vi "MGCC_StaEst_main_HTB.vi"() -> ()   [LabVIEW 2016]
doc: "This VI is designed for the state estimation function block. The current version is designed for IEEE13node system. The advanced model will be available in the latest version. There is no input for this VI. Bascially, the input right now comes from the cvs in IEEE13 folder."
uses:
  Finite State Machine/Sub-VIs/MGCC_FntStaMach_gobal.vi
  <vilib>/imath/engines/lvmath2/RunTimeEngine/IndexRead/NIMS M(S,$).vi
  <instcachedir>/0/NIMS M(S,$)_F24F360562DE41D8BE234322A2E15C65.lvgen/NIMS M(S,$)_F24F360562DE41D8BE234322A2E15C65_000.vi
  <vilib>/imathl/engines/lvmath/Functions/Error Handling/Create Error.vi
  <vilib>/imath/engines/lvmath2/RunTimeEngine/BuiltInFunctions/length/NIMS_length(GV).vi
  <instcachedir>/0/NIMS_length(GV)_08A3D13377FD4E4B96F5795FBF3698FA.lvgen/NIMS_length(GV)_08A3D13377FD4E4B96F5795FBF3698FA_000.vi
  <vilib>/imath/engines/lvmath2/RunTimeEngine/RangeToken/NIMS_Range_R3 - Integer.vi
  <instcachedir>/0/NIMS_Range_R3 - Integer_A435E2FF893B4C718FD5055FE39FE2F6.lvgen/NIMS_Range_R3 - Integer_A435E2FF893B4C718FD5055FE39FE2F6_000.vi
  <vilib>/imath/engines/lvmath2/RunTimeEngine/CommandStatement/MC_CommandStatement_break.vi
  <vilib>/imath/engines/lvmath2/RunTimeEngine/IndexRead/NIMS V(S).vi
  <instcachedir>/0/NIMS V(S)_0488751826AF41519A22953C041130DC.lvgen/NIMS V(S)_0488751826AF41519A22953C041130DC_000.vi
  <vilib>/imath/engines/lvmath2/RunTimeEngine/IndexReplace/NIMS V(S)=S.vi
  <instcachedir>/0/NIMS V(S)=S_57E16554CB8B4B90AAB163894F717546.lvgen/NIMS V(S)=S_57E16554CB8B4B90AAB163894F717546_000.vi
  <vilib>/imath/engines/lvmath2/RunTimeEngine/NodeEndStatement/NIMS_NodeEndStatement_Output.vi
  <instcachedir>/0/NIMS_NodeEndStatement_Output_53EC0D466D134D7ABD903AC30B43404B.lvgen/NIMS_NodeEndStatement_Output_53EC0D466D134D7ABD903AC30B43404B_005.vi
  <vilib>/imath/engines/lvmath2/RunTimeEngine/ErrorHandling/NIMS_Finalize Error.vi
  <vilib>/Utility/error.llb/Error Cluster From Error Code.vi
  Sub-VIs/MGCC_StaEst_global.vi
  Model Management/Global_MdlMgmt.vi
  Abnormal Fault State Control/Sub_VIs/Fault_Abnormal_state.vi
  <vilib>/ErrorRing/Error Ring.xnode
panel:
  in  "Boolean":bool
  out "st_MGCC_StaEst_Input":T1
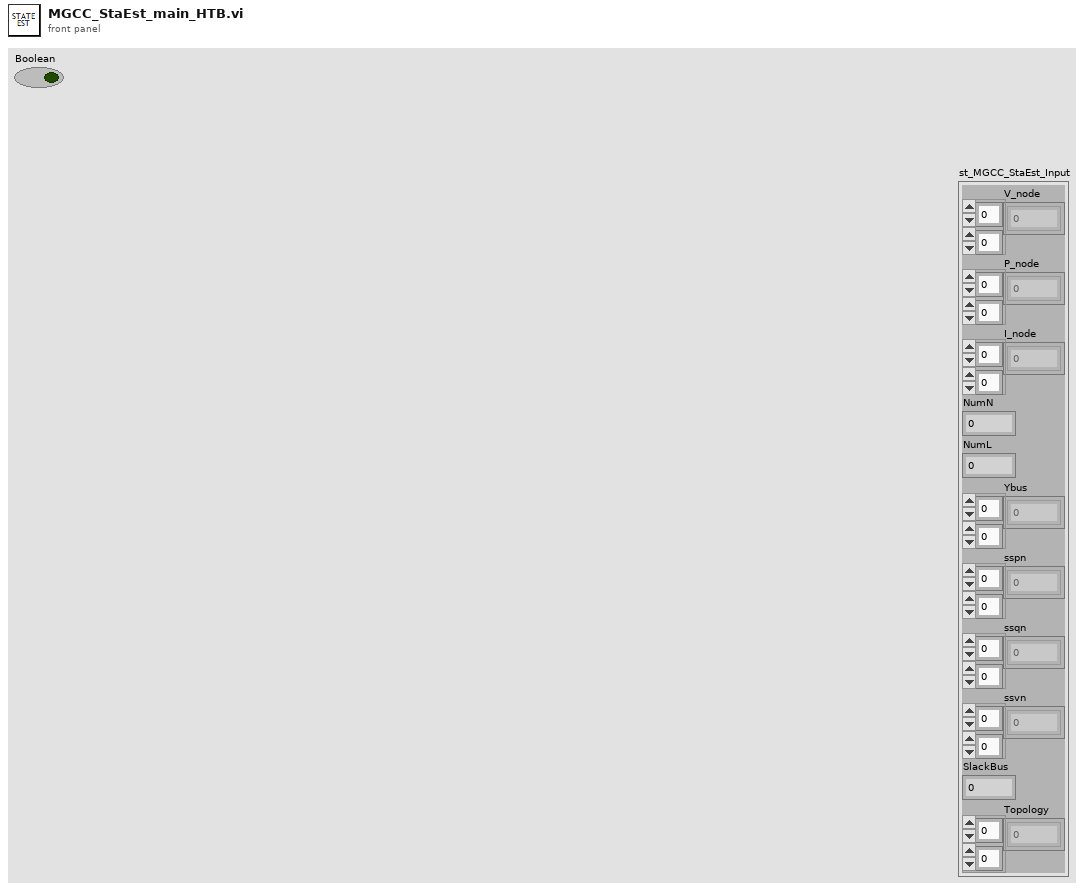
[diagram p1: front panel]
types:
  T1 = cluster{"V_node":cdb[][], "P_node":cdb[][], "I_node":cdb[][], "NumN":dbl, "NumL":dbl, "Ybus":cdb[][], "sspn":dbl[][], "ssqn":dbl[][], "ssvn":dbl[][], "SlackBus":dbl, "Topology":dbl[][]}
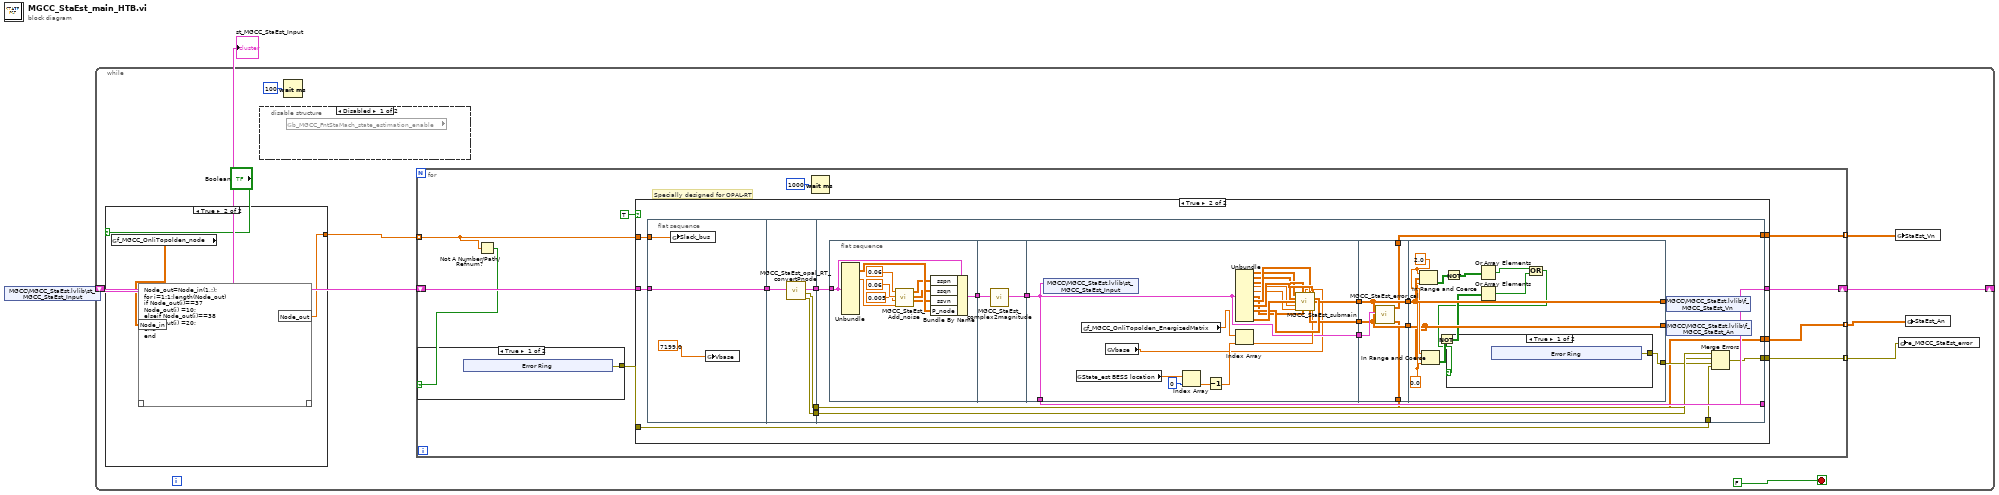
[diagram p0: block diagram]
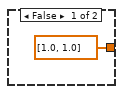
[diagram p2: hidden frame]
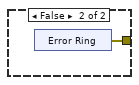
[diagram p3: hidden frame]
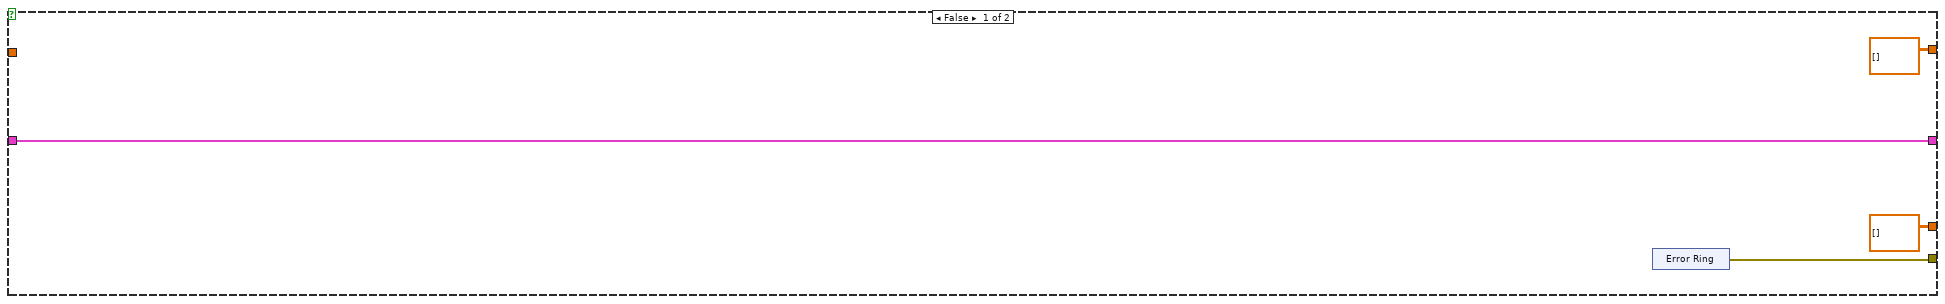
[diagram p4: hidden frame]
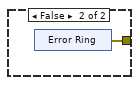
[diagram p5: hidden frame]
diagram:
  n1 = shared-variable "MGCC\\MGCC_StaEst.lvlib\\st_MGCC_StaEst_Input"() -> (w1:T1)  [unwired: 1 in, 1 out]
  "st_MGCC_StaEst_Input" <- w1
  n2 = while {
    shift-right: [w8] -> _
    shift-left: w1 -> [w9]
    stop <- FALSE stop-if-true
    n3 = case shown="True" "Boolean" {
      tunnel: [dbl[] [1.0, 1.0] ("f_MGCC_OnliTopolden_node") w13] -> w4
      frame False {
      }
      frame True {
        n4 = global read "MGCC_FntStaMach_gobal.vi" "f_MGCC_OnliTopolden_node"() -> (w12:dbl[][])
        n5 = mathscript code="Node_out=Node_in(1,:);\nfor i=1:1:length(Node_out)\nif Node_out(i)==37\nNode_out(i) =10;\nelseif Node_out(i)==38\nNode_out(i) =20;\nend\nend"("Node_in"=w12) -> ("Node_out"=w13:dbl[])  [unwired: 1 in, 1 out]
      }
    }
    n6 = disable-structure shown="Disabled" {
      frame Disabled {
        n7 = global read "MGCC_FntStaMach_gobal.vi" "b_MGCC_FntStaMach_state_estimation_enable"() -> ()  [unwired: 1 out]
      }
      frame Enabled {
      }
    }
    n8 = Wait (ms)(milliseconds to wait=u32 100) -> ()  [unwired: 1 out]
    n9 = for {
      shift-right: [w193] -> w8
      shift-left: w9 -> [w194]
      tunnel: w4 -> [w189] mode=indexing
      tunnel: [w190] -> w7 mode=indexing
      tunnel: [w186] -> w3 mode=indexing
      tunnel: [w185] -> w2 mode=indexing
      # "Specially designed for OPAL-RT"
      n10 = Not A Number/Path/Refnum?(number/path/refnum=w189) -> (NaN/Path/Refnum?=w188:bool)
      n11 = case shown="True" w188 {
        tunnel: [w195 w201] -> w187
        frame True {
          n12 = xnode "Error Ring"() -> ("error out"=w195:errorcluster)
        }
        frame False {
          n13 = xnode "Error Ring"() -> ("error out"=w201:errorcluster)
        }
      }
      n14 = case shown="True" TRUE {
        tunnel: w194 -> [w206 w217]
        tunnel: [w206 w216] -> w193
        tunnel: w189 -> [_ w215]
        tunnel: [w205 w213] -> w190
        tunnel: w187 -> [_ w210]
        tunnel: [dbl[][] [] ("output_Vn") w209] -> w186
        tunnel: [dbl[][] [] ("output_An") w208] -> w185
        frame False {
          n15 = xnode "Error Ring"() -> ("error out"=w205:errorcluster)
        }
        frame True {
          n16 = flat-sequence {
            tunnel: w215 -> [w220]
            tunnel: w217 -> [w221]
            tunnel: [w221] -> w214
            tunnel: [w225] -> w218
            tunnel: w214 -> [w224]
            tunnel: [w223] -> w212
            tunnel: [w222] -> w211
            tunnel: w218 -> [w237]
            tunnel: [w233] -> w216
            tunnel: [w232] -> w213
            tunnel: w212 -> [w231]
            tunnel: w211 -> [w230]
            tunnel: w210 -> [w228]
            tunnel: [w227] -> w209
            tunnel: [w226] -> w208
            frame #0 {
              n17 = global write "MGCC_StaEst_global.vi" "Slack_bus"(w220) -> ()
              n18 = global write "MGCC_StaEst_global.vi" "Vbase"(7199.0) -> ()
            }
            frame #1 {
              n19 = call "MGCC_StaEst_opal_RT_convertPnode.vi"("cluster"=w224) -> ("error out 2"=w223:errorcluster, "error out 3"=w222:errorcluster, "P_node"=w225:T1)  [unwired: 8 in]
            }
            frame #2 {
              n20 = flat-sequence {
                tunnel: w237 -> [w252]
                tunnel: [w251] -> w236
                tunnel: w236 -> [w254]
                tunnel: [w255] -> w235
                tunnel: [w266] -> w243
                tunnel: [w265] -> w242
                tunnel: w235 -> [w260]
                tunnel: [w260] -> w234
                tunnel: [w260] -> w233
                tunnel: [w279] -> w241
                tunnel: w243 -> [w279]
                tunnel: [w278] -> w240
                tunnel: w242 -> [w278]
                tunnel: w234 -> [w280]
                tunnel: [w277] -> w227
                tunnel: [w276] -> w226
                tunnel: [w292] -> w239
                tunnel: [w289] -> w238
                tunnel: w241 -> [w292]
                tunnel: w240 -> [w289]
                tunnel: [w281] -> w229
                frame #0 {
                  n21 = Unbundle(w252) -> ("P_node"=w253:cdb[][], "NumN"=w244:dbl)  [unwired: 9 out]
                  n22 = call "MGCC_StaEst_Add_noise.vi"("spn"=0.06, "sqn"=0.06, "svn"=0.005, "Node"=w244) -> ("sspn"=w250:dbl[][], "ssvn"=w249:dbl[][], "ssqn"=w248:dbl[][])  [unwired: 2 in]
                  n23 = Bundle By Name(cluster=w252, "sspn"=w250, "ssqn"=w249, "ssvn"=w248, "P_node"=w253) -> (w251:T1)
                }
                frame #1 {
                  n24 = call "MGCC_StaEst_complex2magnitude.vi"("st_MGCC_StaEst_Input"=w254) -> ("output cluster"=w255:T1)  [unwired: 10 in]
                }
                frame #2 {
                  n25 = shared-variable "MGCC\\MGCC_StaEst.lvlib\\st_MGCC_StaEst_Input"(w260) -> ()  [unwired: 1 in, 1 out]
                  n26 = global read "Global_MdlMgmt.vi" "State_est BESS location"() -> (w263:dbl[])
                  n27 = global read "MGCC_FntStaMach_gobal.vi" "f_MGCC_OnliTopolden_EnergizedMatrix"() -> (w256:dbl[])
                  n28 = global read "MGCC_StaEst_global.vi" "Vbase"() -> (w257:dbl)
                  n29 = Index Array(array=w263, index=0) -> (element=w259:dbl)
                  n30 = Decrement(x=w259) -> (x-1=w258:dbl)
                  n31 = Unbundle(w260) -> ("V_node"=w267:cdb[][], "P_node"=w264:cdb[][], "I_node"=w268:cdb[][], "NumN"=w269:dbl, "NumL"=w270:dbl, "Ybus"=w271:cdb[][], "sspn"=w272:dbl[][], "ssqn"=w273:dbl[][], "ssvn"=w274:dbl[][], "Topology"=w275:dbl[][])  [unwired: 1 out]
                  n32 = Index Array(array=w256, index=w258) -> (element=w261:dbl)
                  n33 = call "MGCC_StaEst_submain.vi"("V_node"=w267, "I_node"=w268, "vbase"=w257, "sspn"=w272, "ssqn"=w273, "P_node"=w264, "ssvn"=w274, "Topology"=w275, "NumN"=w269, "NumL"=w270, "Ybus"=w271, "interrupt"=w261) -> ("VN"=w266:dbl[][], "AN"=w265:dbl[][])  [unwired: 1 in, 1 out]
                }
                frame #3 {
                  n34 = call "MGCC_StaEst_error_cal.vi"("f_MGCC_StaEst_An"=w278, "f_MGCC_StaEst_Vn"=w279, "cluster"=w280) -> ("output_An"=w276:dbl[][], "output_Vn"=w277:dbl[][])  [unwired: 5 in, 2 out]
                }
                frame #4 {
                  w290 = 0.0
                  w291 = 2.0
                  n35 = In Range and Coerce(upper limit=w291, x=w292, lower limit=w290) -> (In Range?=w288:bool[][])  [unwired: 1 out]
                  n36 = In Range and Coerce(upper limit=w291, x=w289, lower limit=w290) -> (In Range?=w287:bool[][])  [unwired: 1 out]
                  n37 = Not(x=w287) -> (.not. x?=w285:bool[][])
                  n38 = Not(x=w288) -> (.not. x?=w286:bool[][])
                  n39 = Or Array Elements(Boolean array=w286) -> (logical OR=w284:bool)
                  n40 = Or Array Elements(Boolean array=w285) -> (logical OR=w283:bool)
                  n41 = Compound Arithmetic op=OR(w284, w283) -> (w282:bool)
                  n42 = case shown="True" w282 {
                    tunnel: [w293 w299] -> w281
                    frame True {
                      n43 = xnode "Error Ring"() -> ("error out"=w293:errorcluster)
                    }
                    frame False {
                      n44 = xnode "Error Ring"() -> ("error out"=w299:errorcluster)
                    }
                  }
                }
              }
              n45 = shared-variable "MGCC\\MGCC_StaEst.lvlib\\f_MGCC_StaEst_Vn"(w239) -> ()  [unwired: 1 in, 1 out]
              n46 = shared-variable "MGCC\\MGCC_StaEst.lvlib\\f_MGCC_StaEst_An"(w238) -> ()  [unwired: 1 in, 1 out]
              n47 = Merge Errors(w231, w230, w229, w228) -> (w232:errorcluster)
            }
          }
        }
      }
      n48 = Wait (ms)(milliseconds to wait=u32 1000) -> ()  [unwired: 1 out]
    }
    n49 = global write "MGCC_StaEst_global.vi" "StaEst_Vn"(w3) -> ()
    n50 = global write "Fault_Abnormal_state.vi" "e_MGCC_StaEst_error"(w7) -> ()
    n51 = global write "MGCC_StaEst_global.vi" "StaEst_An"(w2) -> ()
  }
